vi "Event Stop.vi"(8 "error in":errorcluster) -> (0 "error out":errorcluster)   [LabVIEW 2024, in "VS Tracing API.lvlib"]
doc: "Records the end of the currently active event on the current timed structure thread.\nThis VI closes the event started by <i>Event Start</i>, calculates and display the event duration.\n\n<b>Parameters</b>\nNone.\n\n<b>Notes</b>\n• Should be called after a matching <i>Event Start</i>.\n• The elapsed time between <i>Event Start</i> and <i>Event Stop</i> is displayed as an event duration in the trace."
uses:
  VS Tracing API.lvlib
  libvs_perfetto.dll
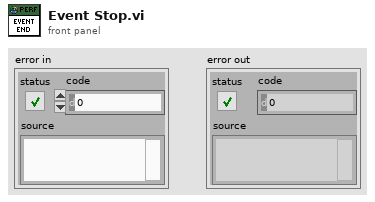
[diagram p1: front panel]
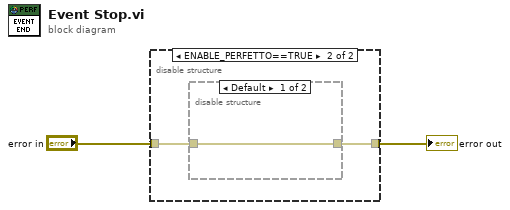
[diagram p0: block diagram]
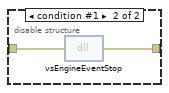
[diagram p3: hidden frame]
diagram:
  n1 = disable-structure shown="ENABLE_PERFETTO==TRUE" {
    disable-tunnel: "error in" -> [w3 w4]
    disable-tunnel: [w3 w5] -> w1
    frame condition #0 (active) {
    }
    frame condition #1 {
      n2 = disable-structure shown="Default" {
        disable-tunnel: [w6 w7] -> w5
        disable-tunnel: w4 -> [w6 w8]
        frame condition #0 (active) {
        }
        frame condition #1 {
          n3 = dll-call lib="libvs_perfetto.*" fn="vsEngineEventStop"(error in=w8) -> (error out=w7:errorcluster)  [unwired: 3 in, 1 out]
        }
      }
    }
  }
  "error out" <- w1
